vi "SQL build mulit data statement.vi"(6 "Equal":string(combo)="=", 8 "error in (no error)":errorcluster, 9 "and/or":string(combo)="or", 10 "ColumnName":string, 11 "ValueArray":string[](array[string])) -> (0 "error out":errorcluster, 3 "concatenated string":string)   [LabVIEW 2021]
doc: "build mulit value statement;"
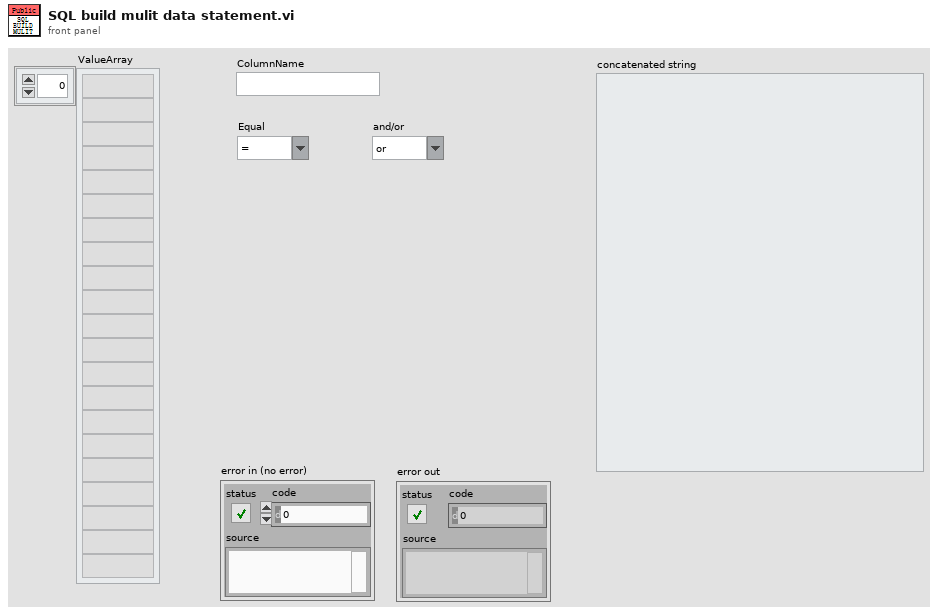
[diagram p1: front panel]
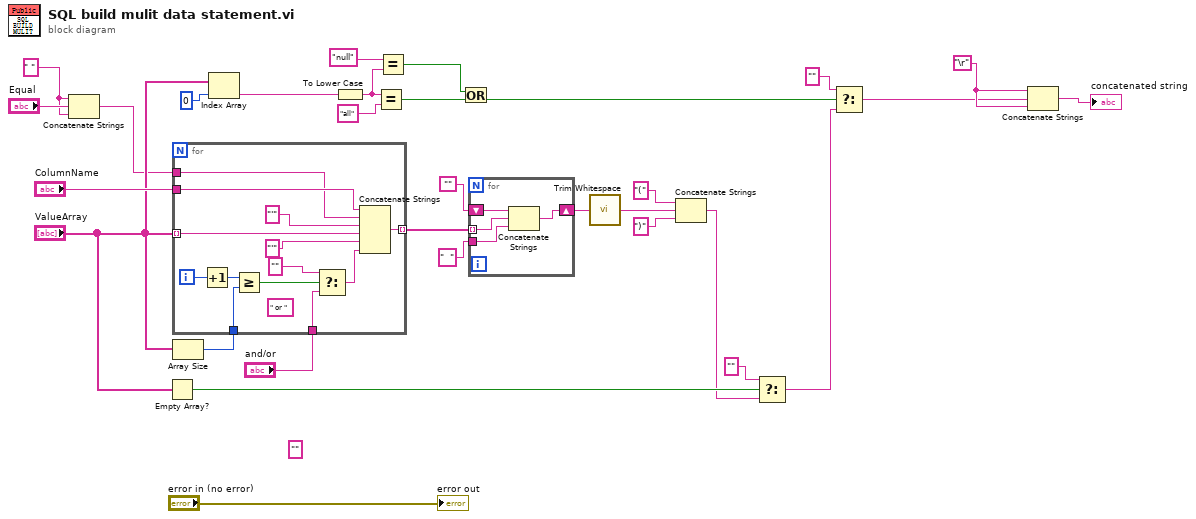
[diagram p0: block diagram]
diagram:
  (unwired) "" ("string")
  w6 = " " ("string")
  w11 = "\r"
  n1 = Concatenate Strings(w6, "Equal", w6) -> (w7:string)
  n2 = Empty Array?(array="ValueArray") -> (empty?=w15:bool)
  n3 = Array Size(array="ValueArray") -> (size(s)=w25:i32)
  n4 = for {
    tunnel: "ValueArray" -> [w44] mode=indexing
    tunnel: [w41] -> w29 mode=indexing
    tunnel: w25 -> [w39]
    tunnel: "ColumnName" -> [w34]
    tunnel: w7 -> [w33]
    tunnel: "and/or" -> [w32]
    i -> [w40]
    (unwired) " or " ("string")
    n5 = Increment(x=w40) -> (x+1=w38:i32)
    n6 = Greater Or Equal?(x=w38, y=w39) -> (x >= y?=w37:bool)
    n7 = Select(t="" ("string"), s=w37, f=w32) -> (s? t:f=w35:string)
    n8 = Concatenate Strings(w34, w33, "'" ("string"), w44, "'" ("string"), w35) -> (w41:string)
  }
  n9 = Index Array(array="ValueArray", index=0) -> (element=w19:string)
  n10 = To Lower Case(string=w19) -> (all lower case string=w4:string)
  n11 = Equal?(x=w4, y="all") -> (x = y?=w21:bool)
  n12 = Equal?(x="null" ("y"), y=w4) -> (x = y?=w2:bool)
  n13 = Or(x=w2, y=w21) -> (x .or. y?=w3:bool)
  n14 = for {
    tunnel: w29 -> [w47] mode=indexing
    shift-right: [w45] -> w26
    shift-left: "" -> [w48]
    tunnel: "  " -> [w46]
    n15 = Concatenate Strings(w48, w47, w46) -> (w45:string)
  }
  n16 = call <vilib>:"Trim Whitespace.vi"("string"=w26) -> ("trimmed string"=w30:string)  [unwired: 1 in]
  n17 = Concatenate Strings("(" ("string"), w30, ")" ("string")) -> (w14:string)
  n18 = Select(t="", s=w15, f=w14) -> (s? t:f=w13:string)
  n19 = Select(t="" ("y"), s=w3, f=w13) -> (s? t:f=w9:string)
  n20 = Concatenate Strings(w11, w9, w11) -> (→"concatenated string":string)
  "error out" <- "error in (no error)"
